vi "ClassPanel.vi"(8 "error in (no error)":errorcluster caption="entrée d'erreur (pas d'erreur)", 11 "AttoAMC300.lvclass":refnum<class "AttoANC300.lvclass">) -> (0 "error out":errorcluster caption="sortie d'erreur", 3 "AttoAMC300.lvclass Out":refnum<class "AttoANC300.lvclass">)   [LabVIEW 2019, in "AttoANC300.lvclass"]
uses:
  AttoANC300.lvclass
  C:/Programmes Labview/LabscanV1A/DevicesClass/BaseDevice/BaseDevice.lvclass
  AttoANC300_Func.ctl
  AttoANC300.lvclass/AttoANC300.ctl
  BaseDevice/ClassQueueMess.ctl
  BaseDevice/BaseDevice.lvclass/BaseDevice.ctl
  BaseDevice/Accessor/SetShowInstrNm.vi
  BaseDevice/Accessor/GetClassEvent.vi
  <userlib>/AMC300/AMC_VIs.lvlib
panel:
  out "ControlsNames":string[](array[string])
  in  "AttoAMCTab":enum32{"Main", "Settings", "RES/Adv"}(tab)
  in  "QuickPan":bool caption="MiseAJour"
  in  "Ctrl loop":bool
  in  "Enable":bool
  in  "Con/Disc.":bool
  out "ActPos":dbl=60.0 caption="Actual Pos(um)" min=0.1 step=0.1 format="%#.3f"
  in  "Read\nCont.":bool
  out "Moving":bool
  in  "Fast\nScan":bool
  out "ActVoltage":i32=60 caption="Act.Volt(mv)" min=1 step=1
  out "In Rng":bool
  out "FWD Lim":bool caption="FWD\nLim"
  out "BKD Lim":bool caption="BKD\nLim"
  in  "Target":dbl=60.0 caption="Target(um)" min=-25000.0 max=25000.0 step=0.001 format="%#.3f"
  in  "Target Rng":dbl=60.0 caption="Tgt Rng.(nm)" min=1.0 step=1.0 format="%#.1f"
  in  "Ampl.(V)":dbl min=0.0 max=60.0 step=0.001
  in  "Freq.(Hz)":dbl=10.0 min=10.0 max=2000.0 step=0.001
  in  "ctrlrange":i32 caption="Ctrl Rng.(nm)"
  in  "TestCap":bool caption="MiseAJour"
  in  "CtrlSens":i32=60 caption="Ctrl Sensitivity" min=1 step=1
  in  "FinePosRng":i32=60 caption="Fine Pos. Rng.(nm)" min=1 step=1
  in  "Refresh(ms)":u32=300
  out "resistance":i32
  out "capacitance":i32
  in  "Gnd On\nTarget":bool
  in  "GndTargetRng":i32=60 caption="Gnd Tgt. Rng.(nm)" min=1 step=1
  out "GND":bool
  in  "Axis":i32(ring) items=["1", "2", "3"]
  out "Axis Model":string
  in  "Reset":bool caption="MiseAJour"
  in  "FinePosSR":i32(ring) caption="Fine Pos SlewRate" items=["Slow", "Slow Medium", "Medium Fast", "Fast"]
  in  "RES Gain":i32(ring) caption="RES Gain (0db 600mv^2/R)" items=["0dB", "-10dB", "-15dB", "-20dB"]
  in  "RES Mode":i32(ring) items=["Individual"=1, "Shared"=2, "Individual LowFreq"=3, "Shared LowFreq"=4]
  in  "Meas Functions":T1
  out "QuickPanRef":refnum<vi>
  in  "MainProgQ":refnum<queue>
  in  "MainProgQEvent":refnum<user-event>
  in  "Acq":bool
  in  "Stop":bool
  out "Init Program":bool
  in  "Axis Name":string
  # "this MUST labeled with class name"
  # "this MUST be present and labeled \"Stop\" and \"Acq\""
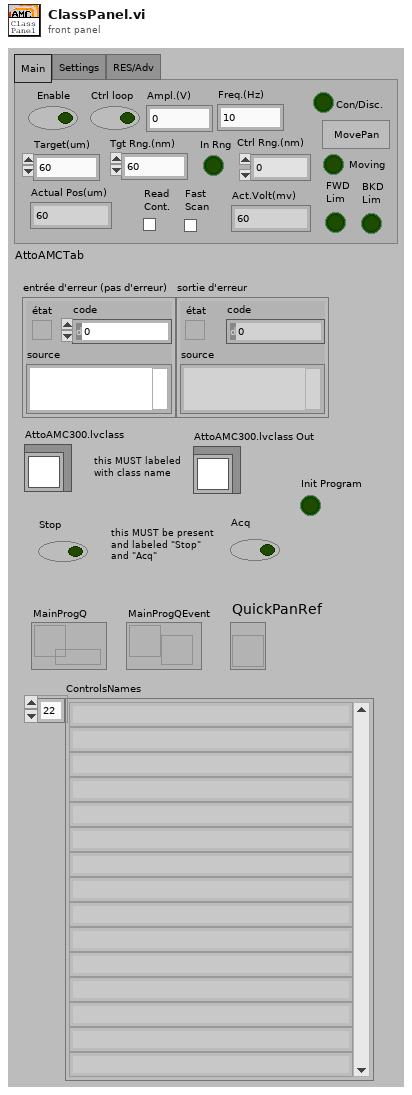
[diagram p1: front panel]
types:
  T1 = typedef "AttoANC300.lvclass/AttoANC300_Func.ctl" = enum16{"MotionMon (um)", "VoltDC (V)"}
  T2 = typedef "ClassQueueMess.ctl" = u16
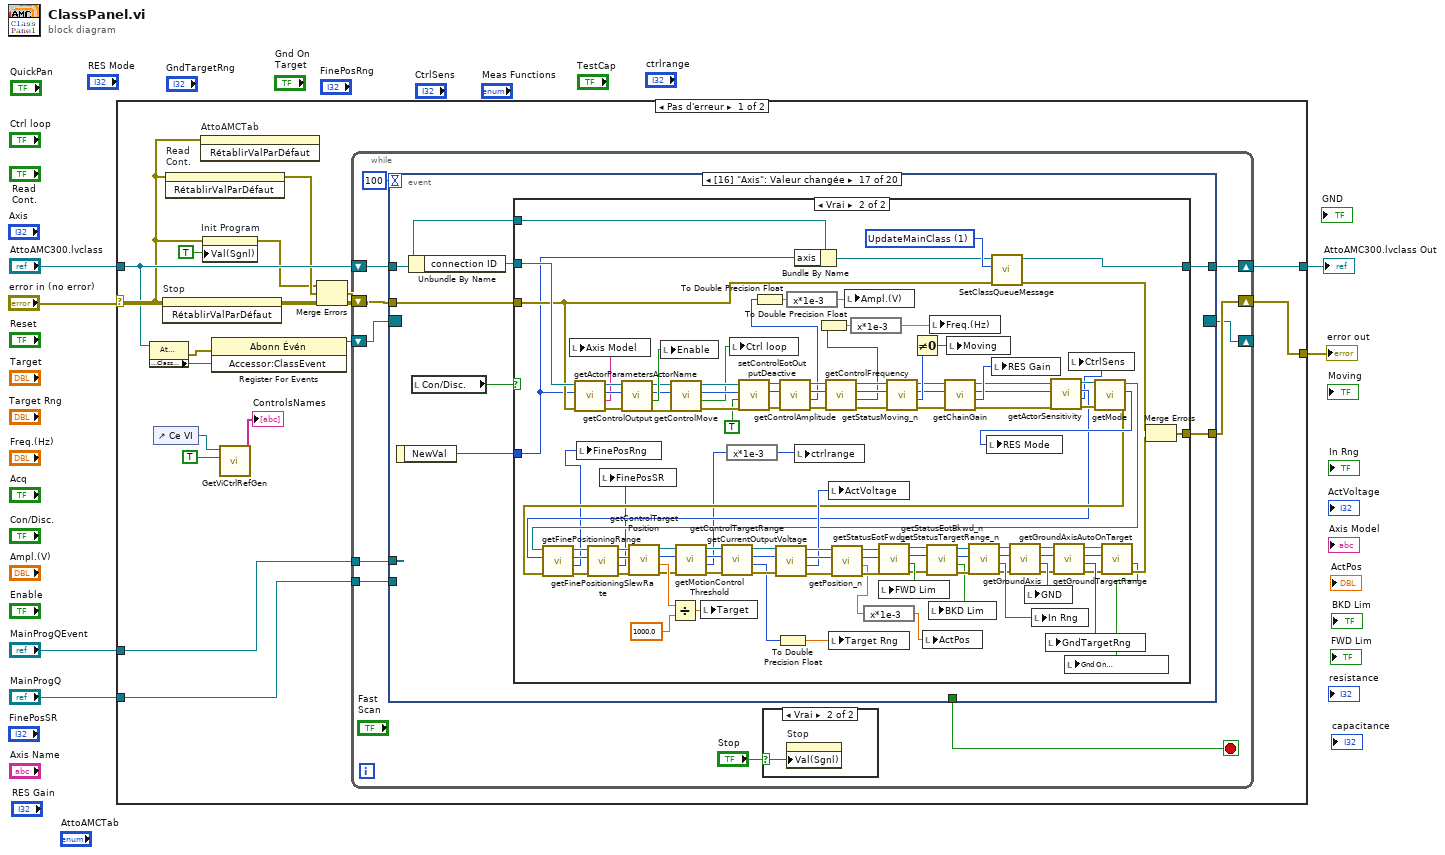
[diagram p0: block diagram]
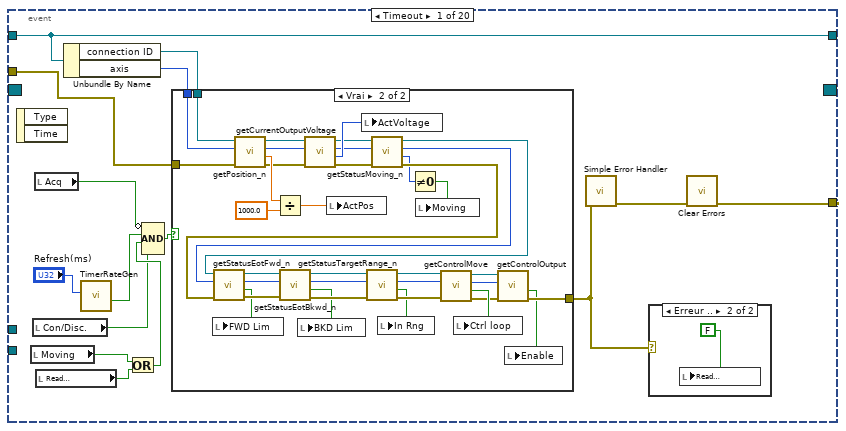
[diagram p3: hidden frame]
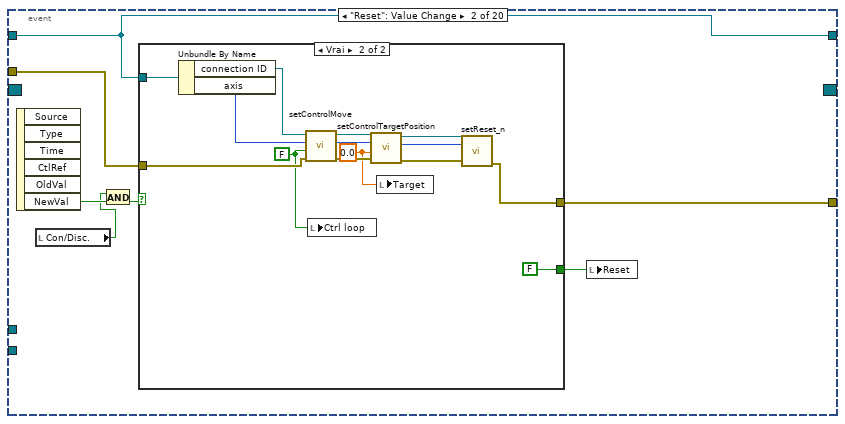
[diagram p6: hidden frame]
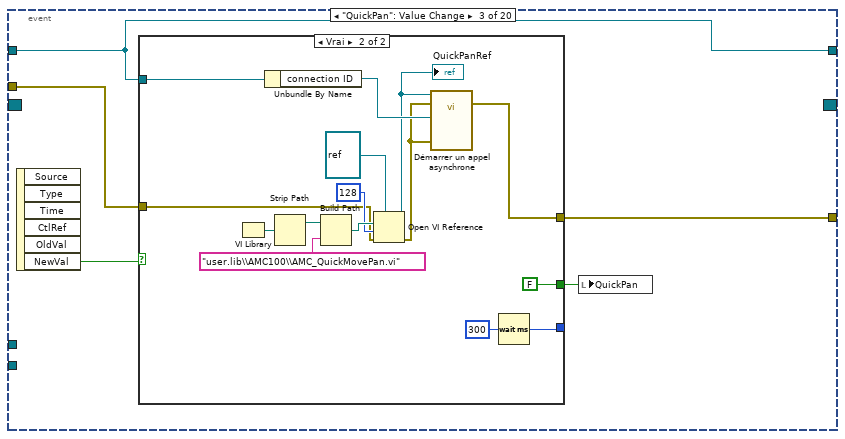
[diagram p8: hidden frame]
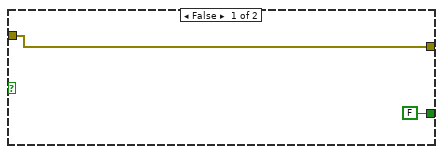
[diagram p9: hidden frame]
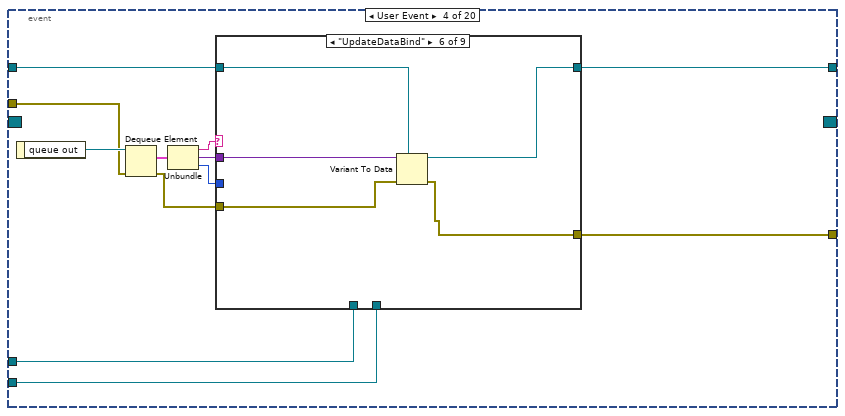
[diagram p10: hidden frame]
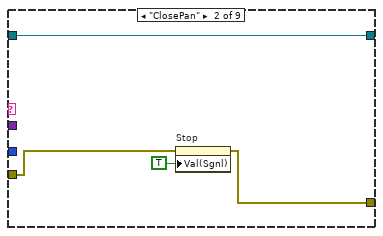
[diagram p12: hidden frame]
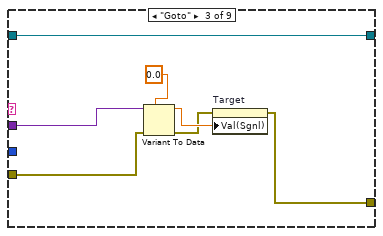
[diagram p13: hidden frame]
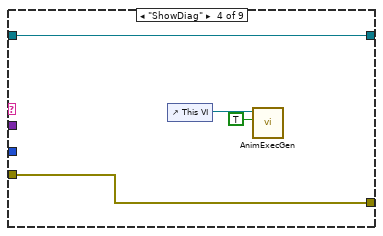
[diagram p14: hidden frame]
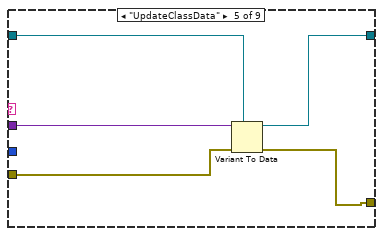
[diagram p15: hidden frame]
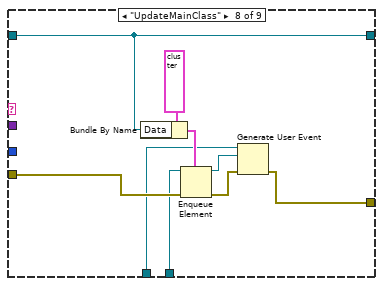
[diagram p17: hidden frame]
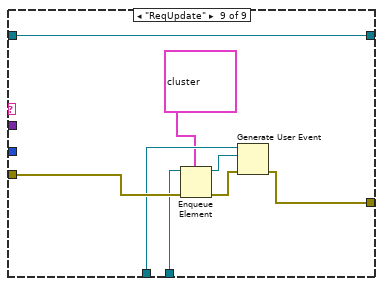
[diagram p18: hidden frame]
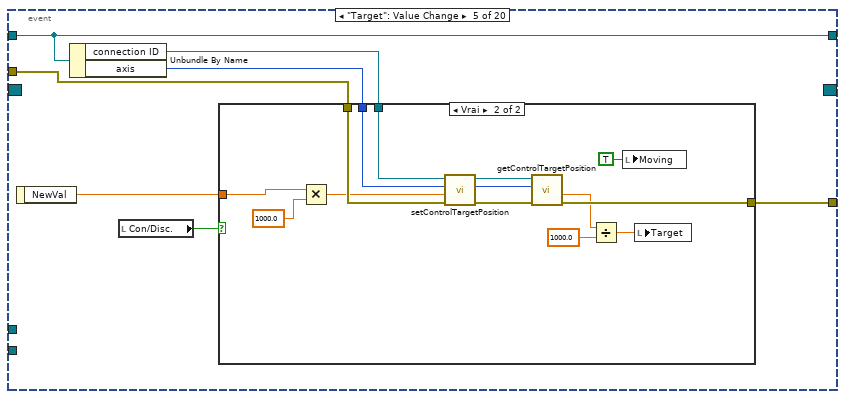
[diagram p19: hidden frame]
diagram:
  n1 = case shown="Pas d'erreur" "error in (no error)" {
    selector: "error in (no error)" -> [w7 w642]
    tunnel: [w23 w642] -> w5
    tunnel: "AttoAMC300.lvclass" -> [w18 w641]
    tunnel: [w22 w641] -> w3
    tunnel: "MainProgQEvent" -> [w16 _]
    tunnel: "MainProgQ" -> [w15 _]
    frame No Error {
      n2 = property class="AttoANC300.lvclass"(reference=w18) -> (error out=w20:errorcluster, "Accessor:ClassEvent"=w19:refnum<user-event>)  [unwired: 1 in, 1 out]
      n3 = control-ref of="Ce VI"() -> (w9:refnum<vi>)
      n4 = invoke on="Stop" class="Bool (strict)" method="RétablirValParDéfaut"(error in=w7) -> (error out=w21:errorcluster)  [unwired: 2 in, 2 out]
      n5 = invoke on="Read\nCont." class="Bool (strict)" method="RétablirValParDéfaut"(error in=w7) -> (error out=w13:errorcluster)  [unwired: 2 in, 2 out]
      n6 = invoke on="AttoAMCTab" class="Onglet (strict)" method="RétablirValParDéfaut"(error in=w7) -> ()  [unwired: 2 in, 3 out]
      n7 = property on="Init Program" class="Bool (strict)"(error in=w7, "Val(Sgnl)"=TRUE ("Valeur (Signalisation)")) -> (error out=w11:errorcluster)  [unwired: 1 in, 1 out]
      n8 = register-events(error in=w20, w19) -> (reference out=w17:refnum<event-registration>)  [unwired: 1 in, 1 out]
      n9 = call <userlib>:"GetViCtrlRefGen.vi"("InclTabCTrl"=TRUE, "VIRef"=w9) -> ("ControlsNames"=→"ControlsNames":string[])  [unwired: 7 in, 2 out]
      n10 = Merge Errors(w11, w13, w21) -> (w14:errorcluster)
      n11 = while {
        shift-right: [w32] -> w23
        shift-left: w14 -> [w33]
        shift-right: [w30] -> w22
        shift-left: w18 -> [w31]
        shift-right: [w28] -> _
        shift-left: w17 -> [w29]
        tunnel: w16 -> [w27]
        tunnel: w15 -> [w26]
        stop <- w24 stop-if-true
        n12 = event shown="[16] \"Axis\": Valeur changée" {
          selector: w29 -> [_ _ _ _ _ _ _ _ _ _ _ _ _ _ _ _ _ _ _ _]
          dyn-events: [_ _ _ _ _ _ _ _ _ _ _ _ _ _ _ _ _ _ _ _] -> w28
          timeout: 100 -> [_ _ _ _ _ _ _ _ _ _ _ _ _ _ _ _ _ _ _ _]
          tunnel: w33 -> [w47 w93 w113 w138 w194 w216 w236 w252 w272 w290 w307 w351 w411 w434 w459 w477 w495 w618 w633 w638]
          tunnel: [w49 w92 w112 w140 w192 w215 w235 w253 w273 w288 w306 w354 w407 w433 w461 w486 w498 w617 w633 _] -> w32
          tunnel: w31 -> [w48 w94 w114 w144 w197 w219 w239 w254 w274 w293 w310 w348 w410 w431 w454 w478 w493 w621 w634 w636]
          tunnel: [_ _ _ _ _ _ _ _ _ _ _ _ _ w432 _ _ _ _ _ _] -> w24
          tunnel: [w48 w94 w114 w139 w197 w219 w239 w254 w274 w293 w310 w348 w409 w431 w460 w488 w497 w621 w634 w636] -> w30
          tunnel: w27 -> [_ _ _ w136 _ _ _ _ _ _ _ _ _ _ _ _ _ _ _ _]
          tunnel: w26 -> [_ _ _ w135 _ _ _ _ _ _ _ _ _ _ _ _ _ _ _ _]
          event Timeout {
            n13 = event-data() -> ()  [unwired: 1 in, 2 out]
            n14 = local read "Moving"() -> (w38:bool)
            n15 = local read "Con/Disc."() -> (w36:bool)
            n16 = local read "Acq"() -> (w41:bool)
            n17 = local read "Read\nCont."() -> (w39:bool)
            n18 = Unbundle By Name(w48) -> ("connection ID"=w46:refnum<k5>, "axis"=w45:i32)
            n19 = call <userlib>:"TimerRateGen.vi"("Refresh(ms)"="Refresh(ms)") -> ("updated?"=w40:bool)  [unwired: 8 in, 2 out]
            n20 = Or(x=w38, y=w39) -> (x .or. y?=w37:bool)
            n21 = Compound Arithmetic op=AND(invert w41, w40, w37, w36) -> (w42:bool)
            n22 = case shown="Vrai" w42 {
              tunnel: w47 -> [w51 w78]
              tunnel: [w51 w65] -> w44
              tunnel: w46 -> [_ w77]
              tunnel: w45 -> [_ w76]
              frame False {
              }
              frame True {
                n23 = call <userlib>:"getPosition_n.vi"("error in"=w78, "axis"=w76, "connection ID"=w77) -> ("error out"=w60:errorcluster, "position"=w68:dbl, "axis_out"=w56:i32, "connection ID"=w61:refnum<k5>)  [unwired: 5 in]
                n24 = Divide(x=w68, y=1000.0) -> (x/y=w67:dbl)
                n25 = call <userlib>:"getCurrentOutputVoltage.vi"("error in"=w60, "axis"=w56, "connection ID"=w61) -> ("error out"=w74:errorcluster, "amplitude"=w75:i32, "axis_out"=w72:i32, "connection ID"=w73:refnum<k5>)  [unwired: 5 in]
                n26 = local write "ActPos"(w67) -> ()
                n27 = local write "ActVoltage"(w75) -> ()
                n28 = call <userlib>:"getStatusMoving_n.vi"("error in"=w74, "axis"=w72, "connection ID"=w73) -> ("error out"=w59:errorcluster, "status"=w54:i32, "axis_out"=w57:i32, "connection ID"=w58:refnum<k5>)  [unwired: 5 in]
                n29 = call <userlib>:"getStatusEotFwd_n.vi"("error in"=w59, "axis"=w57, "connection ID"=w58) -> ("error out"=w83:errorcluster, "detected"=w52:bool, "axis_out"=w86:i32, "connection ID"=w87:refnum<k5>)  [unwired: 5 in]
                n30 = local write "FWD Lim"(w52) -> ()
                n31 = call <userlib>:"getStatusEotBkwd_n.vi"("error in"=w83, "axis"=w86, "connection ID"=w87) -> ("error out"=w82:errorcluster, "detected"=w53:bool, "axis_out"=w84:i32, "connection ID"=w85:refnum<k5>)  [unwired: 5 in]
                n32 = local write "BKD Lim"(w53) -> ()
                n33 = call <userlib>:"getStatusTargetRange_n.vi"("error in"=w82, "axis"=w84, "connection ID"=w85) -> ("error out"=w79:errorcluster, "in_range"=w71:bool, "axis_out"=w80:i32, "connection ID"=w81:refnum<k5>)  [unwired: 5 in]
                n34 = local write "In Rng"(w71) -> ()
                n35 = Not Equal To 0?(x=w54) -> (x != 0?=w55:bool)
                n36 = local write "Moving"(w55) -> ()
                n37 = call <userlib>:"getControlMove.vi"("error in"=w79, "axis"=w80, "connection ID"=w81) -> ("error out"=w66:errorcluster, "enable"=w70:bool, "axis_out"=w63:i32, "connection ID"=w62:refnum<k5>)  [unwired: 5 in]
                n38 = local write "Ctrl loop"(w70) -> ()
                n39 = call <userlib>:"getControlOutput.vi"("error in"=w66, "axis"=w63, "connection ID"=w62) -> ("error out"=w65:errorcluster, "enabled"=w64:bool)  [unwired: 5 in, 2 out]
                n40 = local write "Enable"(w64) -> ()
              }
            }
            n41 = call <vilib>:"Simple Error Handler.vi"("error in (no error)"=w44) -> ("error out"=w50:errorcluster)  [unwired: 4 in, 4 out]
            n42 = case shown="Erreur .." w44 {
              frame No Error {
              }
              frame Error {
                n43 = local write "Read\nCont."(FALSE ("cas vrai")) -> ()
              }
            }
            n44 = call <vilib>:"Clear Errors.vi"("error in (no error)"=w50) -> ("error out"=w49:errorcluster)  [unwired: 5 in, 1 out]
          }
          event "Reset": Value Change {
            n45 = event-data() -> ("NewVal"=w95:bool)  [unwired: 1 in, 5 out]
            n46 = local read "Con/Disc."() -> (w89:bool)
            n47 = And(x=w89, y=w95) -> (x .and. y?=w90:bool)
            n48 = case shown="Vrai" w90 {
              tunnel: w94 -> [_ w110]
              tunnel: w93 -> [w96 w105]
              tunnel: [w96 w109] -> w92
              tunnel: [_ FALSE] -> w91
              frame False {
              }
              frame True {
                w97 = 0.0 ("Target Position in")
                w98 = FALSE ("control move in")
                n49 = Unbundle By Name(w110) -> ("connection ID"=w107:refnum<k5>, "axis"=w106:i32)
                n50 = call <userlib>:"setControlMove.vi"("error in"=w105, "enable"=w98, "axis"=w106, "connection ID"=w107) -> ("error out"=w104:errorcluster, "axis_out"=w103:i32, "connection ID"=w102:refnum<k5>)  [unwired: 5 in]
                n51 = local write "Ctrl loop"(w98) -> ()
                n52 = call <userlib>:"setControlTargetPosition.vi"("error in"=w104, "target"=w97, "axis"=w103, "connection ID"=w102) -> ("error out"=w101:errorcluster, "axis_out"=w99:i32, "connection ID"=w100:refnum<k5>)  [unwired: 5 in]
                n53 = local write "Target"(w97) -> ()
                n54 = call <userlib>:"setReset_n.vi"("error in"=w101, "axis"=w99, "connection ID"=w100) -> ("error out"=w109:errorcluster)  [unwired: 6 in, 2 out]
              }
            }
            n55 = local write "Reset"(w91) -> ()
          }
          event "QuickPan": Value Change {
            n56 = event-data() -> ("NewVal"=w115:bool)  [unwired: 1 in, 5 out]
            n57 = case shown="Vrai" w115 {
              tunnel: w114 -> [_ w122]
              tunnel: w113 -> [w117 w120]
              tunnel: [w117 w121] -> w112
              tunnel: [FALSE FALSE] -> w111
              tunnel: [_ w119] -> _
              frame False {
              }
              frame True {
                n58 = VI Library() -> (path=w129:path)
                n59 = Unbundle By Name(w122) -> ("connection ID"=w131:refnum<k5>)
                n60 = Strip Path(path=w129) -> (stripped path=w128:path)  [unwired: 1 out]
                n61 = Build Path(base path=w128, name or relative path="user.lib\\AMC100\\AMC_QuickMovePan.vi" ("nom ou chemin relatif")) -> (appended path=w127:path)
                n62 = Open VI Reference(type specifier VI Refnum (for type only)=refnum<vi> refnum ("spécificateur de type du refnum de VI (pour type seulement)"), vi path=w127, options=128, error in (no error)=w120) -> (vi reference=w124:refnum<vi>, error out=w125:errorcluster)  [unwired: 2 in]
                "QuickPanRef" <- w124
                n63 = call-by-ref "Démarrer un appel asynchrone"(reference=w124, error in=w125, 8:"error in (no error)"=w125, "ConnID"=w131) -> (error out=w121:errorcluster)  [unwired: 9 in, 2 out]
                n64 = Wait (ms)(milliseconds to wait=u32 300 ("attente (ms)")) -> (millisecond timer value=w119:u32)
              }
            }
            n65 = local write "QuickPan"(w111) -> ()
          }
          event User Event {
            n66 = event-data() -> ("queue out"=w142:refnum<queue>)  [unwired: 1 in]
            n67 = Dequeue Element(queue=w142, error in (no error)=w138) -> (element=w143:cluster{"Message":string, "Data":variant, i32}, error out=w137:errorcluster)  [unwired: 1 in, 2 out]
            n68 = Unbundle(w143) -> ("Message"=w134:string, "Data"=w141:variant, w133:i32)
            n69 = case shown="\"UpdateDataBind\"" w134 {
              tunnel: w137 -> [w146 w149 w152 w161 w164 w169 w172 w177 w187]
              tunnel: w141 -> [_ _ w156 _ w166 w171 _ _ _]
              tunnel: w144 -> [w145 w150 w157 w160 w165 w170 w173 w178 w188]
              tunnel: [w145 w150 w157 w160 w162 w167 w173 w178 w188] -> w139
              tunnel: [w146 w148 w151 w161 w163 w168 w172 w174 w184] -> w140
              tunnel: w133 -> [_ _ _ _ _ _ _ _ _]
              tunnel: w136 -> [_ _ _ _ _ _ _ w176 w186]
              tunnel: w135 -> [_ _ _ _ _ _ _ w175 w185]
              frame Default {
              }
              frame "ClosePan" {
                n70 = property on="Stop" class="Bool (strict)"(error in=w149, "Val(Sgnl)"=TRUE ("Valeur (Signalisation)")) -> (error out=w148:errorcluster)  [unwired: 1 in, 1 out]
              }
              frame "Goto" {
                n71 = Variant To Data(error in=w152, type=0.0, Variant=w156) -> (data=w154:dbl, error out=w153:errorcluster)
                n72 = property on="Target" class="NumNb (strict)"(error in=w153, "Val(Sgnl)"=w154) -> (error out=w151:errorcluster)  [unwired: 1 in, 1 out]
              }
              frame "ShowDiag" {
                n73 = control-ref of="This VI"() -> (w159:refnum<vi>)
                n74 = call <userlib>:"AnimExecGen.vi"("Animer l'exécution ?"=TRUE, "ViRef"=w159) -> ()  [unwired: 9 in, 1 out]
              }
              frame "UpdateClassData" {
                n75 = Variant To Data(error in=w164, type=w165, Variant=w166) -> (data=w162:refnum<class "AttoANC300.lvclass">, error out=w163:errorcluster)
              }
              frame "UpdateDataBind" {
                n76 = Variant To Data(error in=w169, type=w170, Variant=w171) -> (data=w167:refnum<class "AttoANC300.lvclass">, error out=w168:errorcluster)
              }
              frame "MeasDone" {
              }
              frame "UpdateMainClass" {
                n77 = Bundle By Name(cluster=cluster{"Message":string, "Data":variant, i32} {"Message"="", "Data"=variant, 0} ("élément"), "Data"=w178) -> (w179:cluster{"Message":string, "Data":variant, i32})
                n78 = Enqueue Element(queue=w175, element=w179, error in (no error)=w177) -> (queue out=w182:refnum<queue>, error out=w181:errorcluster)  [unwired: 1 in, 1 out]
                n79 = Generate User Event(user event=w176, event data cluster=w182, error in=w181) -> (error out=w174:errorcluster)  [unwired: 1 in, 1 out]
              }
              frame "ReqUpdate" {
                n80 = Enqueue Element(queue=w185, element=cluster{"Message":string, "Data":variant, i32} {"Message"="ReqUpdate", "Data"=variant, 0} ("élément"), error in (no error)=w187) -> (queue out=w190:refnum<queue>, error out=w189:errorcluster)  [unwired: 1 in, 1 out]
                n81 = Generate User Event(user event=w186, event data cluster=w190, error in=w189) -> (error out=w184:errorcluster)  [unwired: 1 in, 1 out]
              }
            }
          }
          event "Target": Value Change {
            n82 = event-data() -> ("NewVal"=w193:dbl)  [unwired: 1 in]
            n83 = Unbundle By Name(w197) -> ("connection ID"=w196:refnum<k5>, "axis"=w195:i32)
            n84 = local read "Con/Disc."() -> (w191:bool)
            n85 = case shown="Vrai" w191 {
              tunnel: w196 -> [_ w209]
              tunnel: w195 -> [_ w208]
              tunnel: w194 -> [w198 w207]
              tunnel: w193 -> [_ w206]
              tunnel: [w198 w205] -> w192
              frame False {
              }
              frame True {
                n86 = Multiply(x=w206, y=1000.0) -> (x*y=w204:dbl)
                n87 = call <userlib>:"setControlTargetPosition.vi"("error in"=w207, "target"=w204, "axis"=w208, "connection ID"=w209) -> ("error out"=w210:errorcluster, "axis_out"=w211:i32, "connection ID"=w212:refnum<k5>)  [unwired: 5 in]
                n88 = call <userlib>:"getControlTargetPosition.vi"("error in"=w210, "axis"=w211, "connection ID"=w212) -> ("error out"=w205:errorcluster, "position [nm/µdeg]"=w201:dbl)  [unwired: 5 in, 2 out]
                n89 = Divide(x=w201, y=1000.0) -> (x/y=w200:dbl)
                n90 = local write "Moving"(TRUE ("Moving")) -> ()
                n91 = local write "Target"(w200) -> ()
              }
            }
          }
          event "Target Rng": Value Change {
            n92 = event-data() -> ("NewVal"=w213:dbl)  [unwired: 1 in]
            n93 = Unbundle By Name(w219) -> ("connection ID"=w218:refnum<k5>, "axis"=w217:i32)
            n94 = local read "Con/Disc."() -> (w214:bool)
            n95 = case shown="Vrai" w214 {
              tunnel: w218 -> [_ w227]
              tunnel: w217 -> [_ w226]
              tunnel: w216 -> [w220 w225]
              tunnel: [w220 w224] -> w215
              tunnel: w213 -> [_ w222]
              frame False {
              }
              frame True {
                n96 = call <userlib>:"setControlTargetRange.vi"("error in"=w225, "range"=w222, "axis"=w226, "connection ID"=w227) -> ("error out"=w228:errorcluster, "axis_out"=w229:i32, "connection ID"=w230:refnum<k5>)  [unwired: 5 in]
                n97 = call <userlib>:"getControlTargetRange.vi"("error in"=w228, "axis"=w229, "connection ID"=w230) -> ("error out"=w224:errorcluster, "targetrange"=w223:i32)  [unwired: 5 in, 2 out]
                n98 = To Double Precision Float(number=w223) -> (double precision float=w221:dbl)
                n99 = local write "Target Rng"(w221) -> ()
              }
            }
          }
          event "ctrlrange": Value Change {
            n100 = event-data() -> ("NewVal"=w233:i32)  [unwired: 1 in]
            n101 = Unbundle By Name(w239) -> ("connection ID"=w238:refnum<k5>, "axis"=w237:i32)
            n102 = Multiply(x=w233, y=1000) -> (x*y=w232:i32)
            n103 = local read "Con/Disc."() -> (w234:bool)
            n104 = case shown="Vrai" w234 {
              tunnel: w238 -> [_ w245]
              tunnel: w237 -> [_ w244]
              tunnel: w236 -> [w240 w243]
              tunnel: [w240 w241] -> w235
              tunnel: w232 -> [_ w242]
              frame False {
              }
              frame True {
                n105 = call <userlib>:"setMotionControlThreshold.vi"("error in"=w243, "threshold"=w242, "axis"=w244, "connection ID"=w245) -> ("error out"=w241:errorcluster)  [unwired: 5 in, 2 out]
              }
            }
          }
          event "Ampl.(V)": Value Change {
            n106 = event-data() -> ("NewVal"=w249:dbl)  [unwired: 1 in]
            n107 = Unbundle By Name(w254) -> ("connection ID"=w251:refnum<k5>, "axis"=w250:i32)
            n108 = expression code="x*1e3"(w249) -> (w248:dbl)
            n109 = local read "Con/Disc."() -> (w246:bool)
            n110 = To Long Integer(number=w248) -> (32bit integer=w247:i32)
            n111 = case shown="Faux" w246 {
              tunnel: [w255 w263] -> w253
              tunnel: w252 -> [w255 w262]
              tunnel: w251 -> [_ w261]
              tunnel: w250 -> [_ w260]
              tunnel: w247 -> [_ w259]
              frame False {
              }
              frame True {
                n112 = call <userlib>:"setControlAmplitude.vi"("error in"=w262, "amplitude"=w259, "axis"=w260, "connection ID"=w261) -> ("error out"=w264:errorcluster, "axis_out"=w265:i32, "connection ID"=w266:refnum<k5>)  [unwired: 5 in]
                n113 = call <userlib>:"getControlAmplitude.vi"("error in"=w264, "axis"=w265, "connection ID"=w266) -> ("error out"=w263:errorcluster, "amplitude"=w257:i32)  [unwired: 5 in, 2 out]
                n114 = To Double Precision Float(number=w257) -> (double precision float=w258:dbl)
                n115 = expression code="x*1e-3"(w258) -> (w256:dbl)
                n116 = local write "Ampl.(V)"(w256) -> ()
              }
            }
          }
          event "Freq.(Hz)": Value Change {
            n117 = event-data() -> ("NewVal"=w269:dbl)  [unwired: 1 in]
            n118 = Unbundle By Name(w274) -> ("connection ID"=w271:refnum<k5>, "axis"=w270:i32)
            n119 = expression code="x*1e3"(w269) -> (w268:dbl)
            n120 = local read "Con/Disc."() -> (w267:bool)
            n121 = case shown="Vrai" w267 {
              tunnel: [w275 w283] -> w273
              tunnel: w272 -> [w275 w282]
              tunnel: w271 -> [_ w281]
              tunnel: w270 -> [_ w280]
              tunnel: w268 -> [_ w279]
              frame False {
              }
              frame True {
                n122 = call <userlib>:"setControlFrequency.vi"("error in"=w282, "frequency"=w279, "axis"=w280, "connection ID"=w281) -> ("error out"=w284:errorcluster, "axis_out"=w285:i32, "connection ID"=w286:refnum<k5>)  [unwired: 5 in]
                n123 = call <userlib>:"getControlFrequency.vi"("error in"=w284, "axis"=w285, "connection ID"=w286) -> ("error out"=w283:errorcluster, "frequency"=w277:i32)  [unwired: 5 in, 2 out]
                n124 = To Double Precision Float(number=w277) -> (double precision float=w278:dbl)
                n125 = expression code="x*1e-3"(w278) -> (w276:dbl)
                n126 = local write "Freq.(Hz)"(w276) -> ()
              }
            }
          }
          event "Enable": Value Change {
            n127 = event-data() -> ("NewVal"=w289:bool)  [unwired: 1 in]
            n128 = Unbundle By Name(w293) -> ("connection ID"=w292:refnum<k5>, "axis"=w291:i32)
            n129 = local read "Con/Disc."() -> (w287:bool)
            n130 = case shown="Faux" w287 {
              tunnel: w292 -> [_ w300]
              tunnel: w291 -> [_ w299]
              tunnel: w290 -> [w294 w298]
              tunnel: w289 -> [_ w297]
              tunnel: [w294 w296] -> w288
              frame False {
              }
              frame True {
                n131 = call <userlib>:"setControlOutput.vi"("error in"=w298, "enable"=w297, "axis"=w299, "connection ID"=w300) -> ("error out"=w301:errorcluster, "axis_out"=w302:i32, "connection ID"=w303:refnum<k5>)  [unwired: 5 in]
                n132 = call <userlib>:"getControlOutput.vi"("error in"=w301, "axis"=w302, "connection ID"=w303) -> ("error out"=w296:errorcluster, "enabled"=w295:bool)  [unwired: 5 in, 2 out]
                n133 = local write "Enable"(w295) -> ()
              }
            }
          }
          event "Enable": Shortcut Menu Selection (User) {
            n134 = event-data() -> ("ItemTag"=w305:string)  [unwired: 1 in, 3 out]
            n135 = Unbundle By Name(w310) -> ("connection ID"=w309:refnum<k5>, "axis"=w308:i32)
            n136 = local read "Con/Disc."() -> (w304:bool)
            n137 = case shown="Faux" w304 {
              tunnel: w309 -> [_ w316]
              tunnel: w308 -> [_ w315]
              tunnel: w307 -> [w311 w314]
              tunnel: [w311 w313] -> w306
              tunnel: w305 -> [_ w312]
              frame False {
              }
              frame True {
                n138 = case shown="\"EnableAll\"" w312 {
                  tunnel: w316 -> [_ w322 w337]
                  tunnel: w315 -> [_ _ _]
                  tunnel: w314 -> [w317 w321 w336]
                  tunnel: [w317 w320 w335] -> w313
                  frame Default {
                  }
                  frame "EnableAll" {
                    n139 = for {
                      N: 3 -> [_]
                      tunnel: w322 -> [w329]
                      tunnel: [w326] -> w319
                      shift-right: [w327] -> w320
                      shift-left: w321 -> [w328]
                      i -> [w324]
                      n140 = Increment(x=w324) -> (x+1=w325:i32)
                      n141 = call <userlib>:"setControlOutput.vi"("error in"=w328, "enable"=TRUE ("enable output in"), "axis"=w325, "connection ID"=w329) -> ("error out"=w330:errorcluster, "axis_out"=w331:i32, "connection ID"=w332:refnum<k5>)  [unwired: 5 in]
                      n142 = call <userlib>:"getControlOutput.vi"("error in"=w330, "axis"=w331, "connection ID"=w332) -> ("error out"=w327:errorcluster, "enabled"=w326:bool)  [unwired: 5 in, 2 out]
                    }
                    n143 = local write "Enable"(w319) -> ()
                  }
                  frame "DisableAll" {
                    n144 = for {
                      N: 3 -> [_]
                      tunnel: w337 -> [w344]
                      tunnel: [w341] -> w334
                      shift-right: [w342] -> w335
                      shift-left: w336 -> [w343]
                      i -> [w339]
                      n145 = Increment(x=w339) -> (x+1=w340:i32)
                      n146 = call <userlib>:"setControlOutput.vi"("error in"=w343, "enable"=FALSE ("enable output in"), "axis"=w340, "connection ID"=w344) -> ("error out"=w345:errorcluster, "axis_out"=w346:i32, "connection ID"=w347:refnum<k5>)  [unwired: 5 in]
                      n147 = call <userlib>:"getControlOutput.vi"("error in"=w345, "axis"=w346, "connection ID"=w347) -> ("error out"=w342:errorcluster, "enabled"=w341:bool)  [unwired: 5 in, 2 out]
                    }
                    n148 = local write "Enable"(w334) -> ()
                  }
                }
              }
            }
          }
          event "Ctrl loop": Value Change {
            n149 = event-data() -> ("NewVal"=w353:bool)  [unwired: 1 in]
            n150 = Unbundle By Name(w348) -> ("connection ID"=w350:refnum<k5>, "axis"=w352:i32)
            n151 = local read "Con/Disc."() -> (w349:bool)
            n152 = case shown="Vrai" w349 {
              tunnel: [w355 w362] -> w354
              tunnel: w353 -> [_ w356]
              tunnel: w352 -> [_ w360]
              tunnel: w351 -> [w355 w359]
              tunnel: w350 -> [_ w358]
              frame False {
              }
              frame True {
                n153 = case shown="Vrai" w356 {
                  tunnel: [TRUE ("T button?") w369] -> w361
                  tunnel: w360 -> [_ w376]
                  tunnel: w359 -> [w366 w375]
                  tunnel: w358 -> [_ w374]
                  tunnel: [w366 w368] -> w357
                  frame False {
                  }
                  frame True {
                    n154 = call <userlib>:"getControlOutput.vi"("error in"=w375, "axis"=w376, "connection ID"=w374) -> ("error out"=w373:errorcluster, "enabled"=w370:bool, "axis_out"=w371:i32, "connection ID"=w372:refnum<k5>)  [unwired: 5 in]
                    n155 = local write "Enable"(w370) -> ()
                    n156 = case shown="Vrai" w370 {
                      tunnel: w373 -> [w377 w395]
                      tunnel: w372 -> [_ w394]
                      tunnel: w371 -> [_ w393]
                      tunnel: [FALSE TRUE ("Set")] -> w369
                      tunnel: [w377 w381] -> w368
                      frame False {
                        n157 = One Button Dialog(message="Axis is not Enable!") -> ()  [unwired: 1 in, 1 out]
                      }
                      frame True {
                        w385 = 1000.0 ("y")
                        n158 = call <userlib>:"getPosition_n.vi"("error in"=w395, "axis"=w393, "connection ID"=w394) -> ("error out"=w387:errorcluster, "position"=w390:dbl, "axis_out"=w388:i32, "connection ID"=w389:refnum<k5>)  [unwired: 5 in]
                        n159 = Divide(x=w390, y=w385) -> (x/y=w392:dbl)
                        n160 = local write "ActPos"(w392) -> ()
                        n161 = call <userlib>:"setControlTargetPosition.vi"("error in"=w387, "target"=w390, "axis"=w388, "connection ID"=w389) -> ("error out"=w384:errorcluster, "axis_out"=w383:i32, "connection ID"=w382:refnum<k5>)  [unwired: 5 in]
                        n162 = call <userlib>:"getControlTargetPosition.vi"("error in"=w384, "axis"=w383, "connection ID"=w382) -> ("error out"=w381:errorcluster, "position [nm/µdeg]"=w380:dbl)  [unwired: 5 in, 2 out]
                        n163 = Divide(x=w380, y=w385) -> (x/y=w386:dbl)
                        n164 = local write "Target"(w386) -> ()
                      }
                    }
                  }
                }
                n165 = case shown="Vrai" w361 {
                  tunnel: w357 -> [w396 w403]
                  tunnel: w356 -> [_ w402]
                  tunnel: w360 -> [_ w401]
                  tunnel: w358 -> [_ w400]
                  tunnel: [w396 w399] -> w362
                  frame False {
                    n166 = local write "Ctrl loop"(FALSE ("Control loop")) -> ()
                  }
                  frame True {
                    n167 = call <userlib>:"setControlMove.vi"("error in"=w403, "enable"=w402, "axis"=w401, "connection ID"=w400) -> ("error out"=w404:errorcluster, "axis_out"=w405:i32, "connection ID"=w406:refnum<k5>)  [unwired: 5 in]
                    n168 = call <userlib>:"getControlMove.vi"("error in"=w404, "axis"=w405, "connection ID"=w406) -> ("error out"=w399:errorcluster, "enable"=w398:bool)  [unwired: 5 in, 2 out]
                    n169 = local write "Ctrl loop"(w398) -> ()
                  }
                }
                n170 = disable-structure shown="Désactivé" {
                  frame Disabled {
                    n171 = local read "Target"() -> (w364:dbl)
                    n172 = Format Into String(format string="Activating control will move stage to target position: %.3f um" ("message"), w364) -> (resulting string=w365:string)  [unwired: 2 in, 1 out]
                    n173 = Two Button Dialog(message=w365) -> ()  [unwired: 2 in, 1 out]
                  }
                  frame Enabled {
                  }
                }
              }
            }
          }
          event "Axis Name": Shortcut Menu Selection (User) {
            n174 = event-data() -> ("ItemTag"=w408:string)  [unwired: 1 in]
            n175 = case shown="\"ChangeName\"" w408 {
              tunnel: w411 -> [w412 w421]
              tunnel: w410 -> [w413 w419]
              tunnel: [w413 w416] -> w409
              tunnel: [w412 w414] -> w407
              frame Default {
              }
              frame "ChangeName" {
                n176 = call "SaveAxisName"("Enable"=TRUE, "error in (no error)"=w421) -> ("Name"=w418:string, "Save"=w417:bool, "error out"=w415:errorcluster)  [unwired: 15 in]
                n177 = case shown="Vrai" w417 {
                  tunnel: w419 -> [w423 w430]
                  tunnel: w418 -> [_ w424]
                  tunnel: [w423 w428] -> w416
                  tunnel: w415 -> [w422 w427]
                  tunnel: [w422 w425] -> w414
                  frame False {
                  }
                  frame True {
                    w426 = T2 1 items=["UpdateClassData", "UpdateMainClass"] ("Menu déroulant")
                    n178 = Bundle By Name(cluster=w430, "AxisName"=w424) -> (w429:refnum<class "AttoANC300.lvclass">)
                    n179 = local write "Axis Name"(w424) -> ()
                    n180 = call-dynamic "SetClassQueueMessage.vi"("ErrorIn(No Error)"=w427, "Menu déroulant"=w426, "DefaultDev.lvclass"=w429) -> ("sortie d'erreur"=w425:errorcluster, "DefaultDev.lvclass Out"=w428:refnum<class "AttoANC300.lvclass">)  [unwired: 7 in]
                  }
                }
              }
            }
          }
          event "Stop": Value Change {
            n181 = event-data() -> ("NewVal"=w432:bool)  [unwired: 1 in, 5 out]
            n182 = case shown="Vrai" w432 {
              tunnel: w431 -> [_ w444]
              tunnel: w434 -> [w435 w438]
              tunnel: [w435 w437] -> w433
              frame False {
              }
              frame True {
                n183 = local read "QuickPanRef"() -> (w439:refnum<vi>)
                n184 = Unbundle By Name(w444) -> ("connection ID"=w441:refnum<k5>)
                n185 = Not A Number/Path/Refnum?(number/path/refnum=w439) -> (NaN/Path/Refnum?=w440:bool)
                n186 = case shown="Faux" w440 {
                  tunnel: w439 -> [w449 _]
                  tunnel: w438 -> [w448 w450]
                  tunnel: [w446 w450] -> w436
                  frame False {
                    n187 = invoke class="Type d'interface de VI 0" method="ValCmde.Déf"(reference=w449, error in=w448, "Control Name"="Quit" ("Nom de la commande"), "Value"=TRUE) -> (error out=w446:errorcluster)  [unwired: 1 in, 4 out]
                  }
                  frame True {
                  }
                }
                n188 = call <userlib>:"AMC_OpenCloseConn.vi"("Open"=FALSE, "error in"=w438, "ConnID"=w441) -> ("error out"=w443:errorcluster)  [unwired: 7 in, 1 out]
                n189 = Merge Errors(w443, w436) -> (w437:errorcluster)
              }
            }
          }
          event "Init Program": Value Change {
            n190 = event-data() -> ()  [unwired: 1 in, 1 out]
            n191 = Unbundle By Name(w454) -> ("Functions"=w451:T1, "axis"=w456:i32, "AxisName"=w452:string)
            n192 = property class="AttoANC300.lvclass"(reference=w454) -> ("Accessor:VisaRes"=w453:refnum<visa-resource-name>)  [unwired: 1 in, 2 out]
            n193 = call <userlib>:"AMC_OpenCloseConn.vi"("Open"=TRUE, "error in"=w459, "deviceAddress"=w453) -> ("error out"=w455:errorcluster, "connection ID"=w458:refnum<k5>)  [unwired: 7 in]
            n194 = local write "Meas Functions"(w451) -> ()
            n195 = local write "Axis Name"(w452) -> ()
            n196 = case shown="Erreur .." w455 {
              selector: w455 -> [w462 w475]
              tunnel: [w462 w471] -> w461
              tunnel: w454 -> [w467 w476]
              tunnel: [w463 w476] -> w460
              tunnel: w458 -> [w466 _]
              tunnel: w456 -> [w465 w469]
              frame No Error {
                n197 = property on="Axis" class="MDér (strict)"("Val(Sgnl)"=w465) -> ()  [unwired: 2 in, 2 out]
                n198 = Bundle By Name(cluster=w467, "connection ID"=w466) -> (w463:refnum<class "AttoANC300.lvclass">)
                n199 = local write "Con/Disc."(TRUE ("Con/Disc.")) -> ()
                "Init Program" <- FALSE
              }
              frame Error {
                w473 = 1 items=["pas d'exception", "annuler l'erreur", "définir l'erreur"] ("[exception action] (none:0)")
                n200 = local write "Axis"(w469) -> ()
                n201 = call <vilib>:"General Error Handler.vi"("error in (no error)"=w475, "[exception action] (none:0)"=w473, "[exception code]"=5000) -> ("error out"=w472:errorcluster)  [unwired: 8 in, 4 out]
                n202 = local write "Con/Disc."(FALSE ("Con/Disc.")) -> ()
                n203 = call <vilib>:"Clear Errors.vi"("error in (no error)"=w472) -> ("error out"=w471:errorcluster)  [unwired: 5 in, 1 out]
              }
            }
          }
          event Value Change {
            w489 = T2 1 items=["UpdateClassData", "UpdateMainClass"] ("Menu déroulant")
            n204 = event-data() -> ("NewVal"=w485:T1)  [unwired: 1 in, 5 out]
            n205 = case shown="\"MotionMon (um)\"" w485 {
              tunnel: [string[] ["ReqPosition(um)", "DetPos(um)"] string[] ["ReqPosition(um)", "DetPos(um)", "Voltage(mv)", "Moving(True)", "InRange(True)"]] -> w482
              frame "VoltDC (V)", Default {
              }
              frame "MotionMon (um)" {
              }
            }
            n206 = Bundle By Name(cluster=w478, "Functions"=w485) -> (w487:refnum<class "AttoANC300.lvclass">)
            n207 = Array Size(array=w482) -> (size(s)=w484:i32)
            n208 = Initialize Array(TRUE, w484) -> (w481:bool[])
            n209 = property class="AttoANC300.lvclass"(reference=w487, error in=w477, "Accessor:DataNames"=w482, "Accessor:ShowInstrNm"=w481) -> (reference out=w479:refnum<class "AttoANC300.lvclass">, error out=w480:errorcluster)
            n210 = call-dynamic "SetClassQueueMessage.vi"("ErrorIn(No Error)"=w480, "Menu déroulant"=w489, "DefaultDev.lvclass"=w479) -> ("sortie d'erreur"=w486:errorcluster, "DefaultDev.lvclass Out"=w488:refnum<class "AttoANC300.lvclass">)  [unwired: 7 in]
          }
          event "Axis": Value Change {
            n211 = event-data() -> ("NewVal"=w492:i32)  [unwired: 1 in]
            n212 = Unbundle By Name(w493) -> ("connection ID"=w494:refnum<k5>)
            n213 = local read "Con/Disc."() -> (w496:bool)
            n214 = case shown="Vrai" w496 {
              tunnel: [w501 w590] -> w498
              tunnel: w493 -> [w499 w609]
              tunnel: [w500 w611] -> w497
              tunnel: w494 -> [_ w568]
              tunnel: w495 -> [w502 w540]
              tunnel: w492 -> [w503 w539]
              frame False {
                w505 = T2 1 items=["UpdateClassData", "UpdateMainClass"] ("Menu déroulant")
                n215 = Bundle By Name(cluster=w499, "axis"=w503) -> (w504:refnum<class "AttoANC300.lvclass">)
                n216 = call-dynamic "SetClassQueueMessage.vi"("ErrorIn(No Error)"=w502, "Menu déroulant"=w505, "DefaultDev.lvclass"=w504) -> ("sortie d'erreur"=w501:errorcluster, "DefaultDev.lvclass Out"=w500:refnum<class "AttoANC300.lvclass">)  [unwired: 7 in]
              }
              frame True {
                w613 = T2 1 items=["UpdateClassData", "UpdateMainClass"] ("Menu déroulant")
                n217 = call <userlib>:"getActorParametersActorName.vi"("error in"=w540, "axis"=w539, "connection ID"=w568) -> ("error out"=w593:errorcluster, "actorname"=w578:string, "axis_out"=w591:i32, "connection ID"=w592:refnum<k5>)  [unwired: 5 in]
                n218 = local write "Axis Model"(w578) -> ()
                n219 = call <userlib>:"getControlOutput.vi"("error in"=w593, "axis"=w591, "connection ID"=w592) -> ("error out"=w601:errorcluster, "enabled"=w602:bool, "axis_out"=w599:i32, "connection ID"=w600:refnum<k5>)  [unwired: 5 in]
                n220 = local write "Enable"(w602) -> ()
                n221 = call <userlib>:"getControlMove.vi"("error in"=w601, "axis"=w599, "connection ID"=w600) -> ("error out"=w596:errorcluster, "enable"=w594:bool, "axis_out"=w598:i32, "connection ID"=w597:refnum<k5>)  [unwired: 5 in]
                n222 = local write "Ctrl loop"(w594) -> ()
                n223 = call <userlib>:"setControlEotOutputDeactive.vi"("error in"=w596, "enable"=TRUE ("enable EOT in"), "axis"=w598, "connection ID"=w597) -> ("error out"=w604:errorcluster, "axis_out"=w603:i32, "connection ID"=w605:refnum<k5>)  [unwired: 5 in]
                n224 = call <userlib>:"getControlAmplitude.vi"("error in"=w604, "axis"=w603, "connection ID"=w605) -> ("error out"=w606:errorcluster, "amplitude"=w519:i32, "axis_out"=w608:i32, "connection ID"=w607:refnum<k5>)  [unwired: 5 in]
                n225 = To Double Precision Float(number=w519) -> (double precision float=w520:dbl)
                n226 = expression code="x*1e-3"(w520) -> (w518:dbl)
                n227 = Bundle By Name(cluster=w609, "axis"=w539) -> (w612:refnum<class "AttoANC300.lvclass">)
                n228 = call <userlib>:"getControlFrequency.vi"("error in"=w606, "axis"=w608, "connection ID"=w607) -> ("error out"=w589:errorcluster, "frequency"=w515:i32, "axis_out"=w587:i32, "connection ID"=w588:refnum<k5>)  [unwired: 5 in]
                n229 = To Double Precision Float(number=w515) -> (double precision float=w517:dbl)
                n230 = local write "Ampl.(V)"(w518) -> ()
                n231 = expression code="x*1e-3"(w517) -> (w516:dbl)
                n232 = call <userlib>:"getStatusMoving_n.vi"("error in"=w589, "axis"=w587, "connection ID"=w588) -> ("error out"=w556:errorcluster, "status"=w564:i32, "axis_out"=w557:i32, "connection ID"=w558:refnum<k5>)  [unwired: 5 in]
                n233 = Not Equal To 0?(x=w564) -> (x != 0?=w565:bool)
                n234 = local write "Freq.(Hz)"(w516) -> ()
                n235 = call <userlib>:"getChainGain.vi"("error in"=w556, "axis"=w557, "connection ID"=w558) -> ("error out"=w524:errorcluster, "gaincoeff"=w555:i32, "axis_out"=w522:i32, "connection ID"=w523:refnum<k5>)  [unwired: 5 in]
                n236 = local write "Moving"(w565) -> ()
                n237 = call-dynamic "SetClassQueueMessage.vi"("ErrorIn(No Error)"=w540, "Menu déroulant"=w613, "DefaultDev.lvclass"=w612) -> ("sortie d'erreur"=w610:errorcluster, "DefaultDev.lvclass Out"=w611:refnum<class "AttoANC300.lvclass">)  [unwired: 7 in]
                n238 = local write "RES Gain"(w555) -> ()
                n239 = call <userlib>:"getActorSensitivity.vi"("error in"=w524, "axis"=w522, "connection ID"=w523) -> ("error out"=w538:errorcluster, "sensitivity"=w525:i32, "axis_out"=w529:i32, "connection ID"=w526:refnum<k5>)  [unwired: 5 in]
                n240 = local write "CtrlSens"(w525) -> ()
                n241 = call <userlib>:"getMode.vi"("error in"=w538, "connection ID"=w526) -> ("error out"=w530:errorcluster, "mode"=w554:i32, "connection ID"=w531:refnum<k5>)  [unwired: 7 in]
                n242 = call <userlib>:"getFinePositioningRange.vi"("error in"=w530, "axis"=w529, "connection ID"=w531) -> ("error out"=w537:errorcluster, "range"=w527:i32, "axis_out"=w536:i32, "connection ID"=w535:refnum<k5>)  [unwired: 5 in]
                n243 = local write "FinePosRng"(w527) -> ()
                n244 = call <userlib>:"getFinePositioningSlewRate.vi"("error in"=w537, "axis"=w536, "connection ID"=w535) -> ("error out"=w534:errorcluster, "slewrate"=w528:i32, "axis_out"=w532:i32, "connection ID"=w533:refnum<k5>)  [unwired: 5 in]
                n245 = local write "FinePosSR"(w528) -> ()
                n246 = call <userlib>:"getControlTargetPosition.vi"("error in"=w534, "axis"=w532, "connection ID"=w533) -> ("error out"=w514:errorcluster, "position [nm/µdeg]"=w567:dbl, "axis_out"=w513:i32, "connection ID"=w512:refnum<k5>)  [unwired: 5 in]
                n247 = Divide(x=w567, y=1000.0) -> (x/y=w569:dbl)
                n248 = call <userlib>:"getMotionControlThreshold.vi"("error in"=w514, "axis"=w513, "connection ID"=w512) -> ("error out"=w511:errorcluster, "range"=w507:i32, "axis_out"=w509:i32, "connection ID"=w510:refnum<k5>)  [unwired: 5 in]
                n249 = local write "Target"(w569) -> ()
                n250 = call <userlib>:"getControlTargetRange.vi"("error in"=w511, "axis"=w509, "connection ID"=w510) -> ("error out"=w563:errorcluster, "targetrange"=w521:i32, "axis_out"=w561:i32, "connection ID"=w562:refnum<k5>)  [unwired: 5 in]
                n251 = expression code="x*1e-3"(w507) -> (w506:i32)
                n252 = call <userlib>:"getCurrentOutputVoltage.vi"("error in"=w563, "axis"=w561, "connection ID"=w562) -> ("error out"=w586:errorcluster, "amplitude"=w583:i32, "axis_out"=w584:i32, "connection ID"=w585:refnum<k5>)  [unwired: 5 in]
                n253 = To Double Precision Float(number=w521) -> (double precision float=w508:dbl)
                n254 = local write "ctrlrange"(w506) -> ()
                n255 = local write "ActVoltage"(w583) -> ()
                n256 = local write "Target Rng"(w508) -> ()
                n257 = call <userlib>:"getPosition_n.vi"("error in"=w586, "axis"=w584, "connection ID"=w585) -> ("error out"=w581:errorcluster, "position"=w560:dbl, "axis_out"=w580:i32, "connection ID"=w582:refnum<k5>)  [unwired: 5 in]
                n258 = expression code="x*1e-3"(w560) -> (w559:dbl)
                n259 = call <userlib>:"getStatusEotFwd_n.vi"("error in"=w581, "axis"=w580, "connection ID"=w582) -> ("error out"=w577:errorcluster, "detected"=w579:bool, "axis_out"=w574:i32, "connection ID"=w575:refnum<k5>)  [unwired: 5 in]
                n260 = local write "FWD Lim"(w579) -> ()
                n261 = local write "ActPos"(w559) -> ()
                n262 = call <userlib>:"getStatusEotBkwd_n.vi"("error in"=w577, "axis"=w574, "connection ID"=w575) -> ("error out"=w576:errorcluster, "detected"=w571:bool, "axis_out"=w573:i32, "connection ID"=w572:refnum<k5>)  [unwired: 5 in]
                n263 = local write "BKD Lim"(w571) -> ()
                n264 = call <userlib>:"getStatusTargetRange_n.vi"("error in"=w576, "axis"=w573, "connection ID"=w572) -> ("error out"=w553:errorcluster, "in_range"=w570:bool, "axis_out"=w552:i32, "connection ID"=w551:refnum<k5>)  [unwired: 5 in]
                n265 = local write "RES Mode"(w554) -> ()
                n266 = call <userlib>:"getGroundAxis.vi"("error in"=w553, "axis"=w552, "connection ID"=w551) -> ("error out"=w549:errorcluster, "grounded"=w550:bool, "axis_out"=w548:i32, "connection ID"=w547:refnum<k5>)  [unwired: 5 in]
                n267 = local write "GND"(w550) -> ()
                n268 = local write "In Rng"(w570) -> ()
                n269 = call <userlib>:"getGroundTargetRange.vi"("error in"=w549, "axis"=w548, "connection ID"=w547) -> ("error out"=w545:errorcluster, "targetrange"=w546:i32, "axis_out"=w544:i32, "connection ID"=w543:refnum<k5>)  [unwired: 5 in]
                n270 = local write "GndTargetRng"(w546) -> ()
                n271 = call <userlib>:"getGroundAxisAutoOnTarget.vi"("error in"=w545, "axis"=w544, "connection ID"=w543) -> ("error out"=w542:errorcluster, "value"=w541:bool)  [unwired: 5 in, 2 out]
                n272 = local write "Gnd On\nTarget"(w541) -> ()
                n273 = Merge Errors(w610, w542) -> (w590:errorcluster)
              }
            }
          }
          event "TestCap": Value Change {
            n274 = event-data() -> ("NewVal"=w622:bool)  [unwired: 1 in, 5 out]
            n275 = Unbundle By Name(w621) -> ("connection ID"=w620:refnum<k5>, "axis"=w619:i32)
            n276 = local read "Con/Disc."() -> (w615:bool)
            n277 = And(x=w622, y=w615) -> (x .and. y?=w616:bool)
            n278 = case shown="Vrai" w616 {
              tunnel: w620 -> [_ w631]
              tunnel: w619 -> [_ w630]
              tunnel: w618 -> [w623 w629]
              tunnel: [w623 w628] -> w617
              tunnel: [_ FALSE] -> w614
              frame False {
              }
              frame True {
                n279 = call <userlib>:"measureCapacitanceAndResistance.vi"("error in"=w629, "axis"=w630, "connection ID in"=w631) -> ("error out"=w628:errorcluster, "CapRes"=w624:cluster{"capacitance":i32, "resistance":i32})  [unwired: 5 in, 2 out]
                n280 = Unbundle(w624) -> ("capacitance"=w625:i32, "resistance"=w626:i32)
                n281 = local write "capacitance"(w625) -> ()
                n282 = local write "resistance"(w626) -> ()
              }
            }
            n283 = local write "TestCap"(w614) -> ()
          }
          event "Con/Disc.": Value Change {
            n284 = event-data() -> ("NewVal"=w632:bool)  [unwired: 1 in, 5 out]
            n285 = case shown="Vrai" w632 {
              frame False {
              }
              frame True {
                n286 = property on="Init Program" class="Bool (strict)"("Val(Sgnl)"=TRUE ("Valeur (Signalisation)")) -> ()  [unwired: 2 in, 2 out]
              }
            }
          }
          event "FWD Lim", "BKD Lim": Value Change {
            n287 = event-data() -> ("CtlRef"=w640:refnum<vi>, "NewVal"=w637:bool)  [unwired: 1 in, 4 out]
            n288 = property class="Bool (strict)"(reference=w640, error in=w638) -> ("Label.Text"=w639:string)  [unwired: 2 out]
            n289 = case shown="\"BKD Lim\"" w639 {
              tunnel: w637 -> [_ _ _]
              frame Default {
              }
              frame "BKD Lim" {
              }
              frame "FWD Lim" {
              }
            }
          }
        }
        n290 = case shown="Vrai" "Stop" {
          selector: "Stop" -> [_ w35]
          frame False {
          }
          frame True {
            n291 = property on="Stop" class="Bool (strict)"("Val(Sgnl)"=w35) -> ()  [unwired: 2 in, 2 out]
          }
        }
      }
    }
    frame Error {
    }
  }
  "error out" <- w5
  "AttoAMC300.lvclass Out" <- w3
